vi "Set_CCD_temperature_setpoint.vi"(8 "error in":errorcluster, 9 "SensorTemperatureSetPoint (C)":dbl, 11 "camera handle in":u64) -> (0 "error out":errorcluster, 3 "camera handle out":u64)   [LabVIEW 2014, in "PICam.lvlib"]
doc: "Sets the temperature setpoint to the desired value, in Celsius units. Use only value from the valid range, depending on your camera specification!\nAfter setting a new setpoint, you need to call the \"Commit_parameters_to_camera.vi\" to send the new value to the camera!"
uses:
  PICam.lvlib
  Picam32.dll
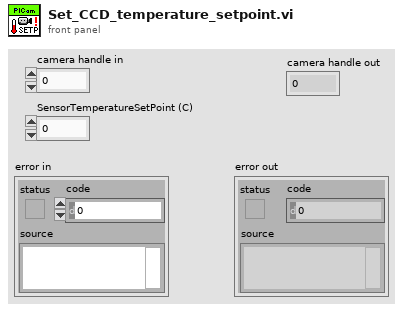
[diagram p1: front panel]
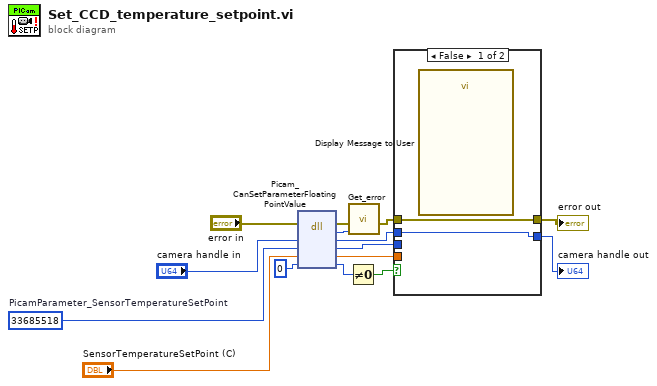
[diagram p0: block diagram]
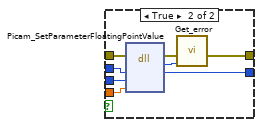
[diagram p2: hidden frame]
diagram:
  w6 = u32 33685518  # PicamParameter_SensorTemperatureSetPoint
  n1 = dll-call lib="Picam32.dll" fn="Picam_CanSetParameterFloatingPointValue"(error in="error in", "camera"="camera handle in", "PicamParameter"=w6, "ExposureTime"="SensorTemperatureSetPoint (C)", "bln"=0 ("CleanSerialRegister")) -> (error out=w14:errorcluster, "return type"=w15:i32, "camera"=w7:u64, "PicamParameter"=w5:u32, "ExposureTime"=w10:dbl, "bln"=w11:i32)  [unwired: 2 in, 1 out]
  n2 = Not Equal To 0?(x=w11) -> (x != 0?=w9:bool)
  n3 = call "Get_error.vi"("PICam_Error"=w15, "error in (no error)"=w14) -> ("error out"=w8:errorcluster)  [unwired: 9 in]
  n4 = case shown="False" w9 {
    tunnel: w10 -> [_ w23]
    tunnel: w8 -> [w17 w22]
    tunnel: w7 -> [w16 w21]
    tunnel: w5 -> [_ w20]
    tunnel: [w17 w19] -> w2
    tunnel: [w16 w18] -> w1
    frame False {
      n5 = call "Display Message to User"() -> ()  [unwired: 10 in, 2 out]
    }
    frame True {
      n6 = dll-call lib="Picam32.dll" fn="Picam_SetParameterFloatingPointValue"(error in=w22, "camera"=w21, "PicamParameter"=w20, "SensorTemperatureSetPoint"=w23) -> (error out=w25:errorcluster, "return type"=w24:i32, "camera"=w18:u64)  [unwired: 4 in, 1 out]
      n7 = call "Get_error.vi"("PICam_Error"=w24, "error in (no error)"=w25) -> ("error out"=w19:errorcluster)  [unwired: 9 in]
    }
  }
  "error out" <- w2
  "camera handle out" <- w1
